vi "Create.vi"(8 "error in (no error)":errorcluster, 9 "Config Folder":path, 10 "Node Config":refnum<class "Node Config.lvclass">, 11 "Volatus Config":refnum<class "VolatusConfig.lvclass">) -> (0 "error out":errorcluster, 3 "VolatusAPI out":refnum<class "VolatusAPI.lvclass">)   [LabVIEW 2020, in "Volatus.lvlib" / "VolatusAPI.lvclass"]
uses:
  VolatusAPI.lvclass
  VolatusConfig/Node/Node Config.lvclass
  C:/dev/lv20CE/relink/lv-volatus/VolatusConfig/VolatusConfigElement/VolatusConfigElement.lvclass
  VolatusConfig/VolatusConfig/VolatusConfig.lvclass
  MsgQs Ref.ctl
  Q Info.ctl
  MessageQ/MessageQ.lvclass
  Registered Q.ctl
  VolatusConfig/VolatusConfigElement/VolatusConfigElement.lvclass/VolatusConfigElement.ctl
  VolatusAPI.lvclass/VolatusAPI.ctl
  VolatusConfig/VolatusConfigElement/Element.vi
  VolatusConfig/VolatusConfigElement/VolatusConfigElement.lvclass
  lv-vecto/Vecto/SubscribedDataHandler/SubscribedDataHandler.lvclass
  C:/dev/lv20CE/relink/lv-volatus/VolatusConfig/Node/Node Config.lvclass
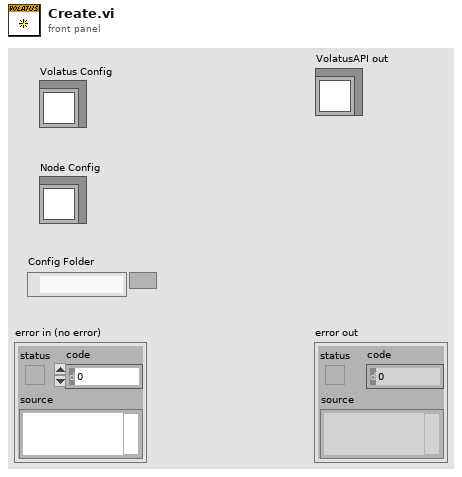
[diagram p1: front panel]
types:
  T1 = map{string, refnum<class "SubscribedDataHandler.lvclass">[]}
  T2 = typedef "Volatus.lvlib/VolatusAPI.lvclass/MsgQs Ref.ctl" = cluster{"Keys":map{string, T3}, "MsgQs":map{i32, T4}, "Next Number":i32}
  T3 = typedef "Volatus.lvlib/VolatusAPI.lvclass/Q Info.ctl" = cluster{"Number":i32, "Notifiers":refnum<notifier>[]}
  T4 = typedef "Volatus.lvlib/VolatusAPI.lvclass/Registered Q.ctl" = cluster{"Q":refnum<class "MessageQ.lvclass">, "Keys":string[]}
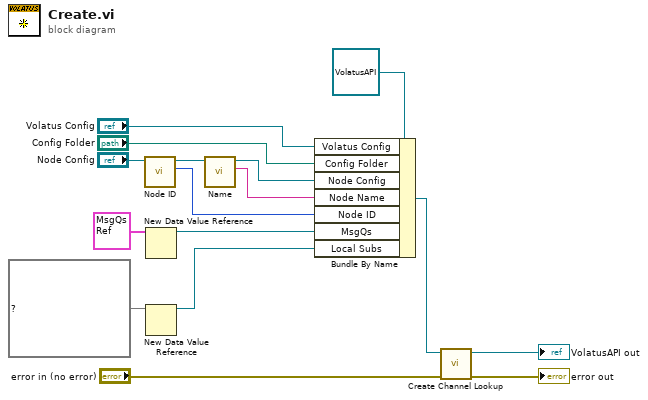
[diagram p0: block diagram]
diagram:
  n1 = call "Node ID.vi"("Node in"="Node Config") -> ("Node ID"=w11:u32, "Node out"=w7:refnum<class "Node Config.lvclass">)  [unwired: 8 in, 1 out]
  n2 = New Data Value Reference(data value=T2 {"Keys"={}, "MsgQs"={}, "Next Number"=0} ("APIs Ref")) -> (data value reference=w13:refnum<data-value>)  [unwired: 1 in, 1 out]
  n3 = New Data Value Reference(data value=T1 {} ("Map")) -> (data value reference=w1:refnum<data-value>)  [unwired: 1 in, 1 out]
  n4 = call "Name.vi"("VolatusConfigElement in"=w7) -> ("Name"=w5:string, "VolatusConfigElement out"=w6:refnum<class "Node Config.lvclass">)  [unwired: 8 in, 1 out]
  n5 = Bundle By Name(cluster=refnum<class "VolatusAPI.lvclass"> refnum ("VolatusAPI in"), "Volatus Config"="Volatus Config", "Config Folder"="Config Folder", "Node Config"=w6, "Node Name"=w5, "Node ID"=w11, "MsgQs"=w13, "Local Subs"=w1) -> (w9:refnum<class "VolatusAPI.lvclass">)
  n6 = call "Create Channel Lookup.vi"("error in (no error)"="error in (no error)", "VolatusAPI in"=w9) -> ("error out"=→"error out":errorcluster, "VolatusAPI out"=→"VolatusAPI out":refnum<class "VolatusAPI.lvclass">)  [unwired: 8 in]
